vi "_nimcDMControlLoop_Subtract(32.16).vi"(2 "Fraction B":i16, 3 "Integer B":i32, 4 "Fraction A":i16, 5 "Integer A":i32) -> (0 "Fraction A-B":u16, 1 "Integer A-B":i32)   [LabVIEW 2014]
doc: "Performs fixed point substraction with both operand in 32.16 format and 32.16 result."
panel:
  # "32.16"
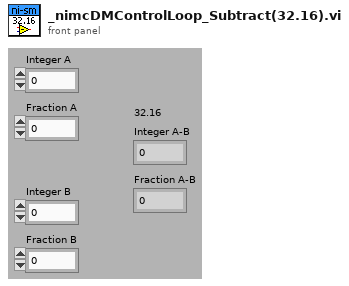
[diagram p1: front panel]
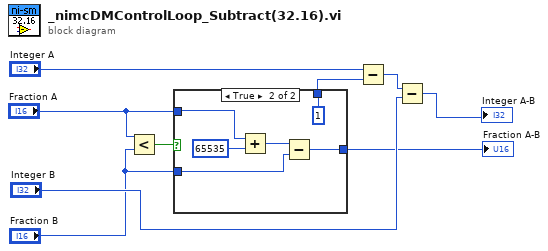
[diagram p0: block diagram]
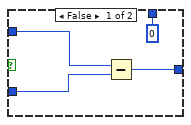
[diagram p2: hidden frame]
diagram:
  n1 = Less?(x="Fraction A", y="Fraction B") -> (x < y?=w9:bool)
  n2 = case shown="True" w9 {
    tunnel: "Fraction B" -> [w12 w15]
    tunnel: "Fraction A" -> [w13 w19]
    tunnel: [w11 w14] -> w1
    tunnel: [0 1] -> w8
    frame False {
      n3 = Subtract(x=w13, y=w12) -> (x-y=w11:i16)
    }
    frame True {
      n4 = Add(x=w19, y=65535) -> (x+y=w16:i32)
      n5 = Subtract(x=w16, y=w15) -> (x-y=w14:i32)
    }
  }
  "Fraction A-B" <- w1
  n6 = Subtract(x="Integer A", y=w8) -> (x-y=w7:i32)
  n7 = Subtract(x=w7, y="Integer B") -> (x-y=→"Integer A-B":i32)
